vi "Refresh Listbox Changes.vi"(8 "error in":errorcluster, 10 "only show changes (T)":bool=TRUE, 11 "refresh listbox":T1[](array[typedef])) -> (0 "error out":errorcluster, 1 "background colors":u32[][](array[colorbox]), 2 "item symbols":T2[](array[typedef])=[enum."Blank", enum."Incoming", enum."Outgoing", enum."Label", enum."Word", enum."Parameter"], 3 "item names":string[][](array[string]))   [LabVIEW 2020, in "Ballard ARINC 429 System Explorer.lvlib" / "Implementation.lvlib"]
doc: "This VI runs when the Add Port run-time menu is chosen. It allows the user to create a port with an associated database."
uses:
  Types/Refresh Symbols.ctl
  Types/Refresh Listbox.ctl
  Implementation.lvlib
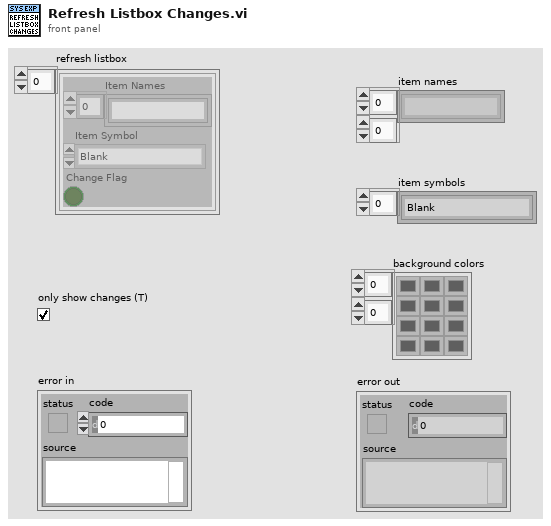
[diagram p1: front panel]
types:
  T1 = typedef "Ballard ARINC 429 System Explorer.lvlib/Implementation.lvlib/Refresh Listbox.ctl" = cluster{"Item Names":string[], "Item Symbol":T2, "Change Flag":bool}
  T2 = typedef "Ballard ARINC 429 System Explorer.lvlib/Implementation.lvlib/Refresh Symbols.ctl" = enum16{"Blank", "Port", "Incoming", "Outgoing", "Label", "Word", "Parameter", "ARINC-429", "Config Files", "Channel Spec", "Item"}
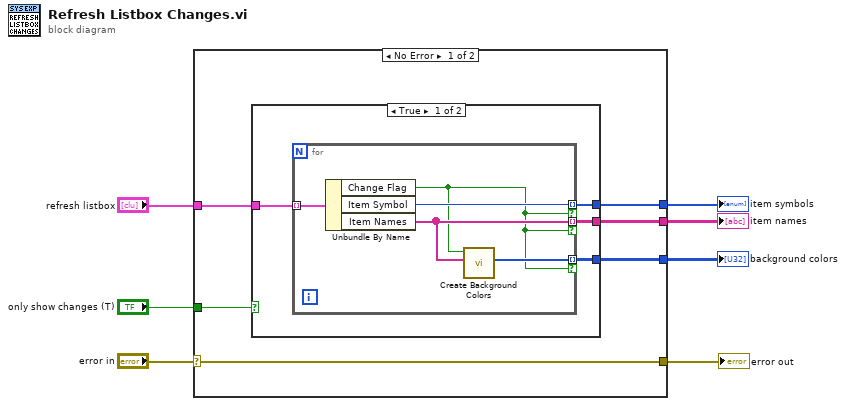
[diagram p0: block diagram]
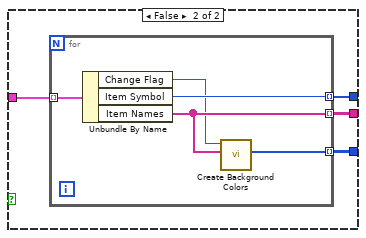
[diagram p2: hidden frame]
diagram:
  n1 = case shown="No Error" "error in" {
    selector: "error in" -> [w10 w32]
    tunnel: "refresh listbox" -> [w9 _]
    tunnel: "only show changes (T)" -> [w13 _]
    tunnel: [w12 _] -> w3
    tunnel: [w11 _] -> w2
    tunnel: [w10 w32] -> w5
    tunnel: [w8 _] -> w1
    frame No Error {
      n2 = case shown="True" w13 {
        tunnel: [w17 w26] -> w12
        tunnel: [w16 w25] -> w11
        tunnel: w9 -> [w15 w24]
        tunnel: [w14 w23] -> w8
        frame True {
          n3 = for {
            tunnel: [w22] -> w17 mode=indexing if=w18
            tunnel: [w19] -> w16 mode=indexing if=w18
            tunnel: w15 -> [w21] mode=indexing
            tunnel: [w20] -> w14 mode=indexing if=w18
            n4 = Unbundle By Name(w21) -> ("Change Flag"=w18:bool, "Item Symbol"=w22:T2, "Item Names"=w19:string[])
            n5 = call "Create Background Colors.vi"("iItem names"=w19, "change flag"=w18) -> ("background colors"=w20:u32[])  [unwired: 9 in]
          }
        }
        frame False {
          n6 = for {
            tunnel: [w31] -> w26 mode=indexing
            tunnel: [w28] -> w25 mode=indexing
            tunnel: w24 -> [w30] mode=indexing
            tunnel: [w29] -> w23 mode=indexing
            n7 = Unbundle By Name(w30) -> ("Change Flag"=w27:bool, "Item Symbol"=w31:T2, "Item Names"=w28:string[])
            n8 = call "Create Background Colors.vi"("iItem names"=w28, "change flag"=w27) -> ("background colors"=w29:u32[])  [unwired: 9 in]
          }
        }
      }
    }
    frame Error {
    }
  }
  "error out" <- w5
  "item names" <- w2
  "item symbols" <- w3
  "background colors" <- w1
